vi "get #OfTests.vi"(8 "error in (no error)":errorcluster caption="Fehler (Eingang, kein Fehler)", 11 "Norm (Eingang)":refnum<class "Norm.lvclass">) -> (0 "error out":errorcluster caption="Fehler (Ausgang)", 2 "#OfTests":u32, 3 "Norm (Ausgang)":refnum<class "Norm.lvclass">)   [LabVIEW 2013, in "DatenKlassen.lvlib" / "Norm.lvclass"]
uses:
  Norm.lvclass
  Norm.lvclass/Norm.ctl
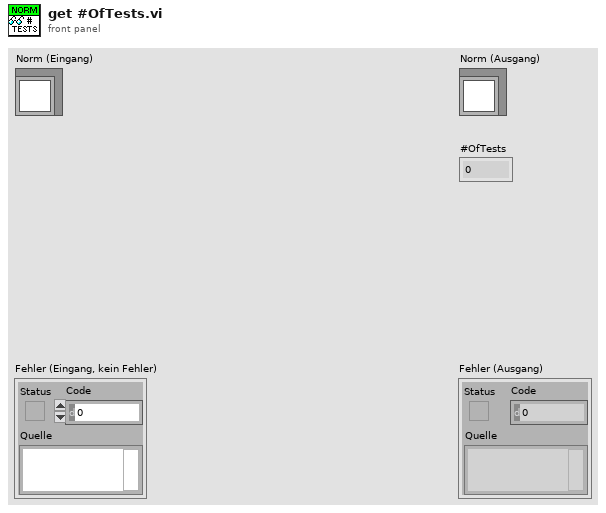
[diagram p1: front panel]
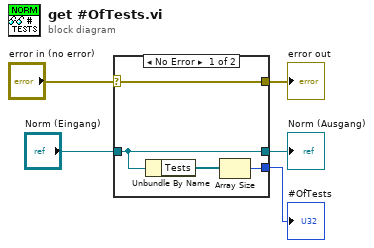
[diagram p0: block diagram]
diagram:
  n1 = case shown="No Error" "error in (no error)" {
    selector: "error in (no error)" -> [w9 w10]
    tunnel: [w9 w10] -> w4
    tunnel: [w8 w11] -> w2
    tunnel: "Norm (Eingang)" -> [w8 w11]
    tunnel: [w6 _] -> w1
    frame No Error {
      n2 = Unbundle By Name(w8) -> ("Tests"=w7:refnum<class "Test.lvclass">[])
      n3 = Array Size(array=w7) -> (size(s)=w6:i32)
    }
    frame Error {
    }
  }
  "error out" <- w4
  "Norm (Ausgang)" <- w2
  "#OfTests" <- w1
